vi "Read Show Buses With Lines.vi"(8 "error in (no error)":errorcluster, 11 "MixedSignalGraph.lvclass in":refnum<class "MixedSignalGraph.lvclass">) -> (0 "error out":errorcluster, 2 "ShowBusesWithLines":bool, 3 "MixedSignalGraph.lvclass out":refnum<class "MixedSignalGraph.lvclass">)   [LabVIEW 2015, in "MixedSignalGraph.lvclass"]
uses:
  MixedSignalGraph.lvclass
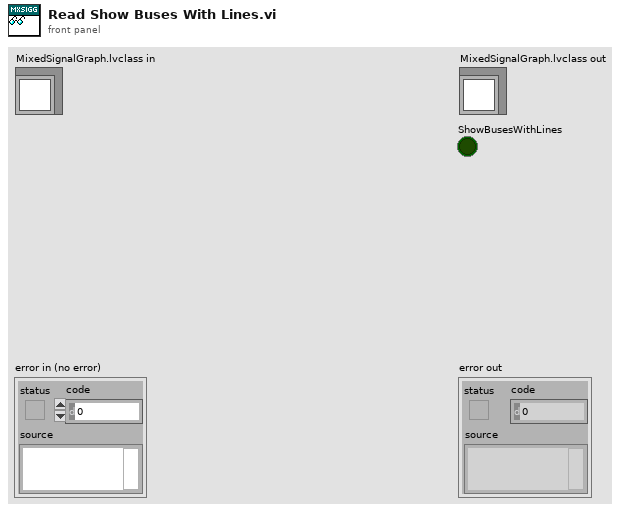
[diagram p1: front panel]
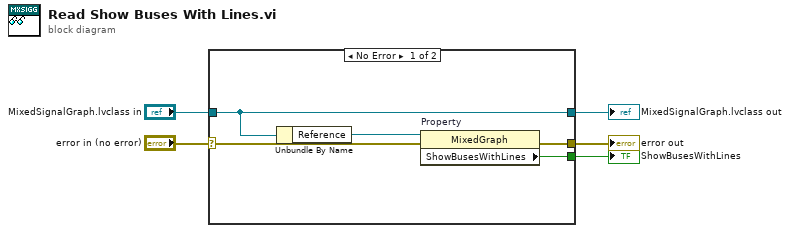
[diagram p0: block diagram]
diagram:
  n1 = case shown="No Error" "error in (no error)" {
    selector: "error in (no error)" -> [w6 w12]
    tunnel: [w9 w12] -> w4
    tunnel: [w8 w11] -> w2
    tunnel: "MixedSignalGraph.lvclass in" -> [w8 w11]
    tunnel: [w10 _] -> w1
    frame No Error {
      n2 = Unbundle By Name(w8) -> ("Reference"=w7:refnum<vi>)
      n3 = property on="Property" class="MixedGraph"(reference=w7, error in=w6) -> (error out=w9:errorcluster, "ShowBusesWithLines"=w10:bool)  [unwired: 1 out]
    }
    frame Error {
    }
  }
  "error out" <- w4
  "MixedSignalGraph.lvclass out" <- w2
  "ShowBusesWithLines" <- w1
